vi "Traffic_Lights_main_v0.vi"() -> ()   [LabVIEW 2020]
uses:
  #typedef_Semaphore.ctl
panel:
  out "West":T1
  out "South":T1
  out "East":T1
  out "North":T1
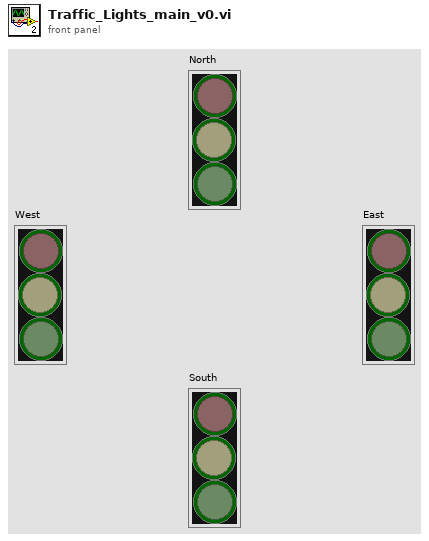
[diagram p1: front panel]
types:
  T1 = typedef "#typedef_Semaphore.ctl" = cluster{"Red":bool, "Yellow":bool, "Green":bool}
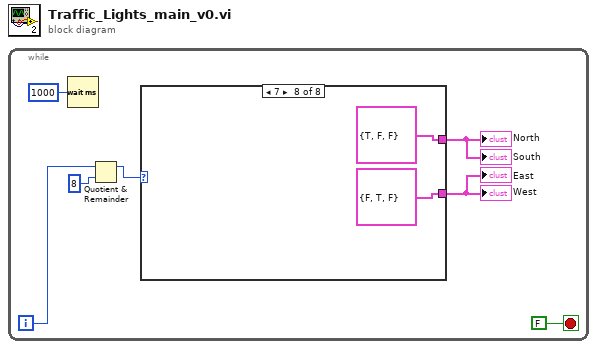
[diagram p0: block diagram]
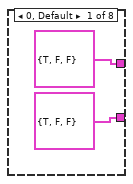
[diagram p2: hidden frame]
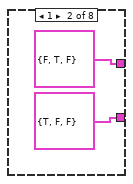
[diagram p3: hidden frame]
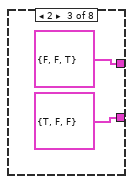
[diagram p4: hidden frame]
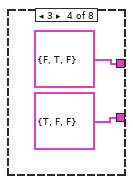
[diagram p5: hidden frame]
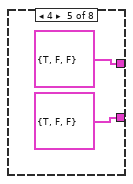
[diagram p6: hidden frame]
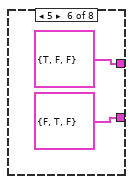
[diagram p7: hidden frame]
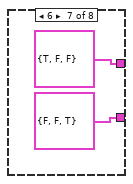
[diagram p8: hidden frame]
diagram:
  n1 = while {
    i -> [w7]
    stop <- FALSE stop-if-true
    n2 = Wait (ms)(milliseconds to wait=u32 1000) -> ()  [unwired: 1 out]
    n3 = Quotient & Remainder(x=w7, y=8) -> (x-y*floor(x/y)=w1:i32)  [unwired: 1 out]
    n4 = case shown="7" w1 {
      tunnel: [T1 {"Red"=TRUE, "Yellow"=FALSE, "Green"=FALSE} ("North") T1 {"Red"=FALSE, "Yellow"=TRUE, "Green"=FALSE} ("North") T1 {"Red"=FALSE, "Yellow"=FALSE, "Green"=TRUE} ("North") T1 {"Red"=FALSE, "Yellow"=TRUE, "Green"=FALSE} ("North") T1 {"Red"=TRUE, "Yellow"=FALSE, "Green"=FALSE} ("North") T1 {"Red"=TRUE, "Yellow"=FALSE, "Green"=FALSE} ("North") T1 {"Red"=TRUE, "Yellow"=FALSE, "Green"=FALSE} ("North") T1 {"Red"=TRUE, "Yellow"=FALSE, "Green"=FALSE} ("North")] -> w6
      tunnel: [T1 {"Red"=TRUE, "Yellow"=FALSE, "Green"=FALSE} ("North") T1 {"Red"=TRUE, "Yellow"=FALSE, "Green"=FALSE} ("North") T1 {"Red"=TRUE, "Yellow"=FALSE, "Green"=FALSE} ("North") T1 {"Red"=TRUE, "Yellow"=FALSE, "Green"=FALSE} ("North") T1 {"Red"=TRUE, "Yellow"=FALSE, "Green"=FALSE} ("North") T1 {"Red"=FALSE, "Yellow"=TRUE, "Green"=FALSE} ("North") T1 {"Red"=FALSE, "Yellow"=FALSE, "Green"=TRUE} ("North") T1 {"Red"=FALSE, "Yellow"=TRUE, "Green"=FALSE} ("North")] -> w5
      frame 0, Default {
      }
      frame 1 {
      }
      frame 2 {
      }
      frame 3 {
      }
      frame 4 {
      }
      frame 5 {
      }
      frame 6 {
      }
      frame 7 {
      }
    }
    "North" <- w6
    "East" <- w5
    "South" <- w6
    "West" <- w5
  }
